vi "BX.Message__LCR.vi"() -> (3 "Messages":T1)   [LabVIEW 2011, in "BooleanXControl__LCR.xctl"]
doc: "Message typedef:\nNone\nEmpty Variant\n\nUsed for a small footpring on the owning BD"
uses:
  BooleanXControl__LCR.xctl
  BX.Message__LCR.ctl
  BX.Commands__LCR.ctl
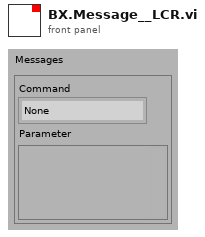
[diagram p1: front panel]
types:
  T1 = typedef "BooleanXControl__LCR.xctl/BX.Message__LCR.ctl" = cluster{"Command":T2, "Parameter":variant}
  T2 = typedef "BooleanXControl__LCR.xctl/BX.Commands__LCR.ctl" = enum16{"None", "SetPicture", "SetFont", "SetText", "SetOrientation", "Redraw", "SetTextColor", "SetRTSettings", "MultipleUpdate", "RT.Button", "RT.Hilite", "RT.Behaviour", "RT.Disabled", "ShowGUI", "RT.Nudge", "RT.Hover", "RT.ButtonType"}
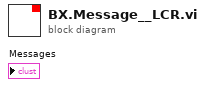
[diagram p0: block diagram]
diagram:
